vi "Set Frequency.vi"(6 "Channel":i32=1, 8 "error in (no error)":errorcluster, 10 "Frequency":dbl, 11 "336XX in":refnum<class "336XX.lvclass">) -> (0 "error out":errorcluster, 3 "336XX out":refnum<class "336XX.lvclass">)   [LabVIEW 2019, in "336XX.lvlib" / "336XX.lvclass"]
uses:
  Library/336XX.lvclass
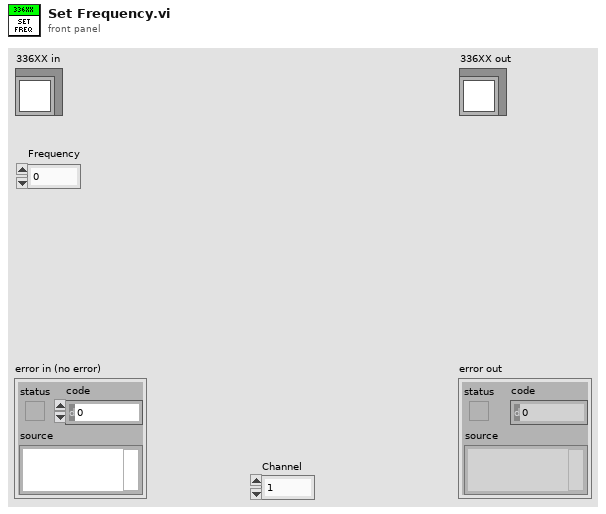
[diagram p1: front panel]
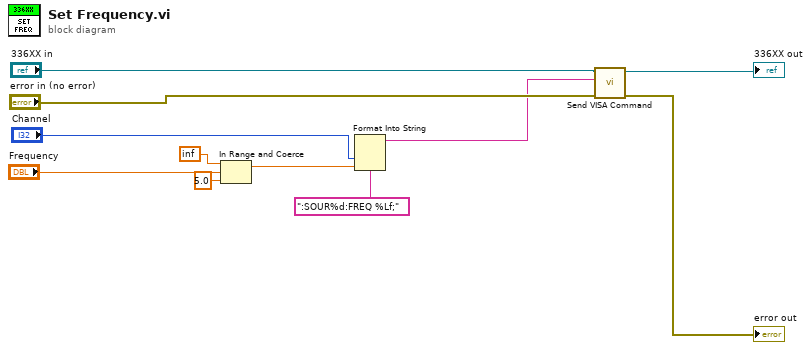
[diagram p0: block diagram]
diagram:
  n1 = In Range and Coerce(upper limit=inf, x="Frequency", lower limit=5.0) -> (coerced(x)=w3:dbl)  [unwired: 1 out]
  n2 = Format Into String(format string=":SOUR%d:FREQ %Lf;", "Channel", w3) -> (resulting string=w2:string)  [unwired: 2 in, 1 out]
  n3 = call "Send VISA Command.vi"("error in (no error)"="error in (no error)", "Command"=w2, "336XX in"="336XX in") -> ("error out"=→"error out":errorcluster, "336XX out"=→"336XX out":refnum<class "336XX.lvclass">)  [unwired: 7 in]
